vi "SendEndofMotionMsg.vi"(5 "Polarization":string, 7 "All Positions, eng units":dbl[](array[numeric]), 8 "error in (no error)":errorcluster, 9 "Move Type":T1, 10 "Position":i32, 11 "SendMessage in":refnum<class "SendMessage.lvclass">) -> (0 "error out":errorcluster, 3 "SendMessage out":refnum<class "SendMessage.lvclass">)   [LabVIEW 2018, in "SendMessage.lvclass"]
doc: "after the end of a motion of long duration, where the service is polling.\nBut could be after the end of any move."
uses:
  SendMessage.lvclass
  VXMMotionManager/MotionTypes.ctl
  Support/MessageAPI/UIMessage.ctl
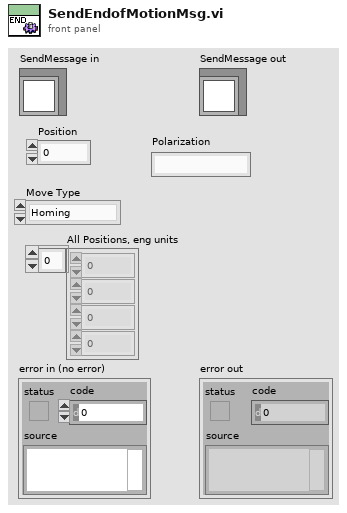
[diagram p1: front panel]
types:
  T1 = typedef "MotionTypes.ctl" = enum16{"Homing", "AllAbsolute", "AllHome", "Position", "OneAxisHome", "Clear"}
  T2 = typedef "UIMessage.ctl" = cluster{"EventCode":i32, "Numeric":dbl, "String":string, "Variant":variant}
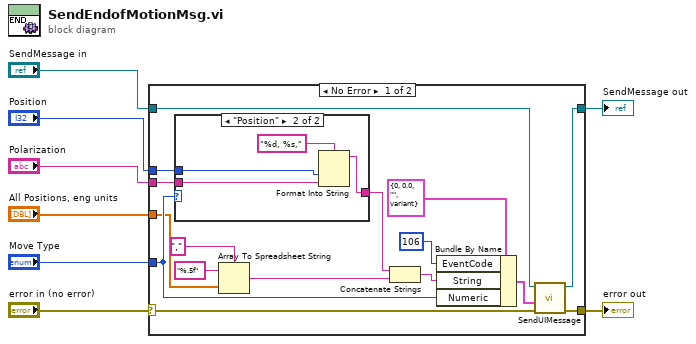
[diagram p0: block diagram]
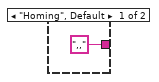
[diagram p2: hidden frame]
diagram:
  n1 = case shown="No Error" "error in (no error)" {
    selector: "error in (no error)" -> [w14 w31]
    tunnel: [w13 w31] -> w7
    tunnel: [w15 w30] -> w5
    tunnel: "SendMessage in" -> [w16 w30]
    tunnel: "Move Type" -> [w12 _]
    tunnel: "All Positions, eng units" -> [w11 _]
    tunnel: "Position" -> [w10 _]
    tunnel: "Polarization" -> [w9 _]
    frame No Error {
      n2 = case shown="\"Position\"" w12 {
        tunnel: w10 -> [_ w29]
        tunnel: [",," w27] -> w24
        tunnel: w9 -> [_ w26]
        frame "Homing", Default {
        }
        frame "Position" {
          n3 = Format Into String(format string="%d, %s,", w29, w26) -> (resulting string=w27:string)  [unwired: 2 in, 1 out]
        }
      }
      n4 = Array To Spreadsheet String(delimiter (Tab)=",", array=w11, 3:"%.5f" ("format string")) -> (spreadsheet string=w22:string)
      n5 = Concatenate Strings(w24, w22) -> (w23:string)
      n6 = Bundle By Name(cluster=T2 {"EventCode"=0, "Numeric"=0.0, "String"="", "Variant"=variant} ("UIMsg"), "EventCode"=106, "String"=w23, "Numeric"=w12) -> (w18:T2)
      n7 = call-dynamic "SendUIMessage.vi"("error in (no error)"=w14, "UIMsg"=w18, "SendMessage in"=w16) -> ("error out"=w13:errorcluster, "SendMessage out"=w15:refnum<class "SendMessage.lvclass">)  [unwired: 7 in]
    }
    frame Error {
    }
  }
  "error out" <- w7
  "SendMessage out" <- w5
